vi "Plugin - Random Data Chart.vi"() -> ()   [LabVIEW 2017]
doc: "Subpanel Plugin VI that displays a random value, multiplied by a user-specified value, in a waveform chart."
panel:
  out "Random Number Chart":dbl(graph)
  in  "Multiplier":dbl(slide)=2.0 scale=0.0..10.0
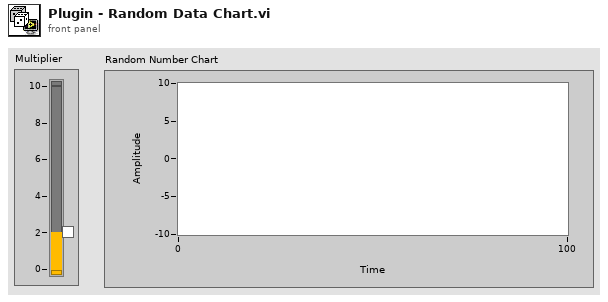
[diagram p1: front panel]
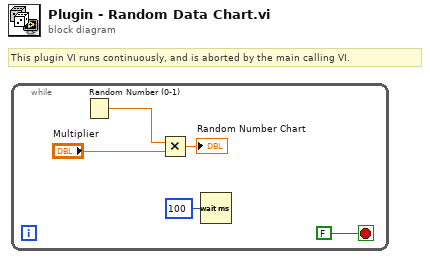
[diagram p0: block diagram]
diagram:
  # "This plugin VI runs continuously, and is aborted by the main calling VI."
  n1 = while {
    stop <- FALSE stop-if-true
    n2 = Random Number (0-1)() -> (number: 0 to 1=w2:dbl)
    n3 = Multiply(x=w2, y="Multiplier") -> (x*y=→"Random Number Chart":dbl)
    n4 = Wait (ms)(milliseconds to wait=u32 100) -> ()  [unwired: 1 out]
  }
